vi "Read State.vi"(8 "error in (no error)":errorcluster, 11 "Cargo in":refnum<class "Cargo.lvclass">) -> (0 "error out":errorcluster, 2 "Enum":T1, 3 "Cargo out":refnum<class "Cargo.lvclass">)   [LabVIEW 2019, in "Cargo.lvlib" / "Cargo.lvclass"]
uses:
  Cargo.lvclass
  Controls/Cargo States.ctl
  Cargo.lvclass/Cargo.ctl
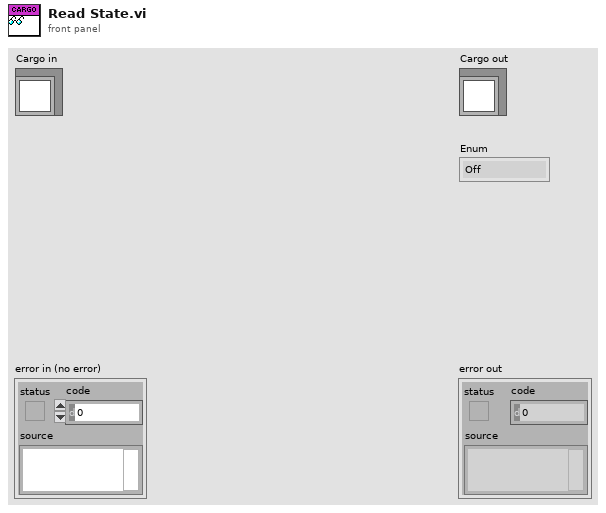
[diagram p1: front panel]
types:
  T1 = typedef "Cargo.lvlib/Cargo.lvclass/Cargo States.ctl" = enum16{"Off", "Intake Full", "Intake Idle", "Output Full"}
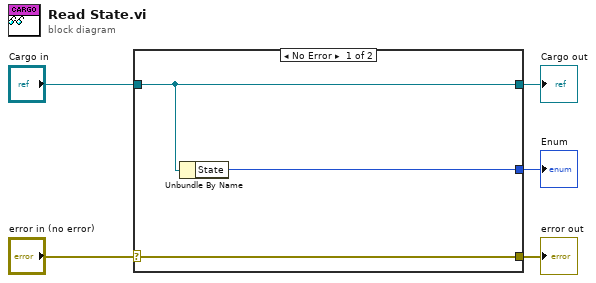
[diagram p0: block diagram]
diagram:
  n1 = case shown="No Error" "error in (no error)" {
    selector: "error in (no error)" -> [w8 w9]
    tunnel: [w8 w9] -> w4
    tunnel: [w7 w10] -> w2
    tunnel: "Cargo in" -> [w7 w10]
    tunnel: [w6 _] -> w1
    frame No Error {
      n2 = Unbundle By Name(w7) -> ("State"=w6:T1)
    }
    frame Error {
    }
  }
  "error out" <- w4
  "Cargo out" <- w2
  "Enum" <- w1
